vi "CLD 10 Step Sequencer with CSV Solution.vi"() -> ()   [LabVIEW 2014]
doc: "CLD-Übung 10\n\nDurch Verwendung des Zustandsautomaten aus CLD 9 und der FGV aus CLD-Übung 6 lässt sich die Entwicklungszeit für diese Übung verkürzen."
uses:
  CLD 10 CSV file read eum.ctl
  CLD 10 CSV file data structure.ctl
  CLD 10 CSV file enum.ctl
panel:
  out "Dauer des aktuellen Schritts":dbl
  out "Verstrichene Zeit (s)":dbl format="%#.2g"
  out "Schritt 3":bool
  out "Schritt 2":bool
  out "Schritt 1":bool
  out "Zeit ist verstrichen":bool
  in  "Autom. zurücksetzen":bool=TRUE
  in  "Zurücksetzen-Schaltfläche":bool
  in  "VI anhalten":bool
  out "Fehler (Ausgang)":errorcluster
  in  "Fehler (Eingang, kein Fehler)":errorcluster
  in  "Zielzeit (s)":dbl
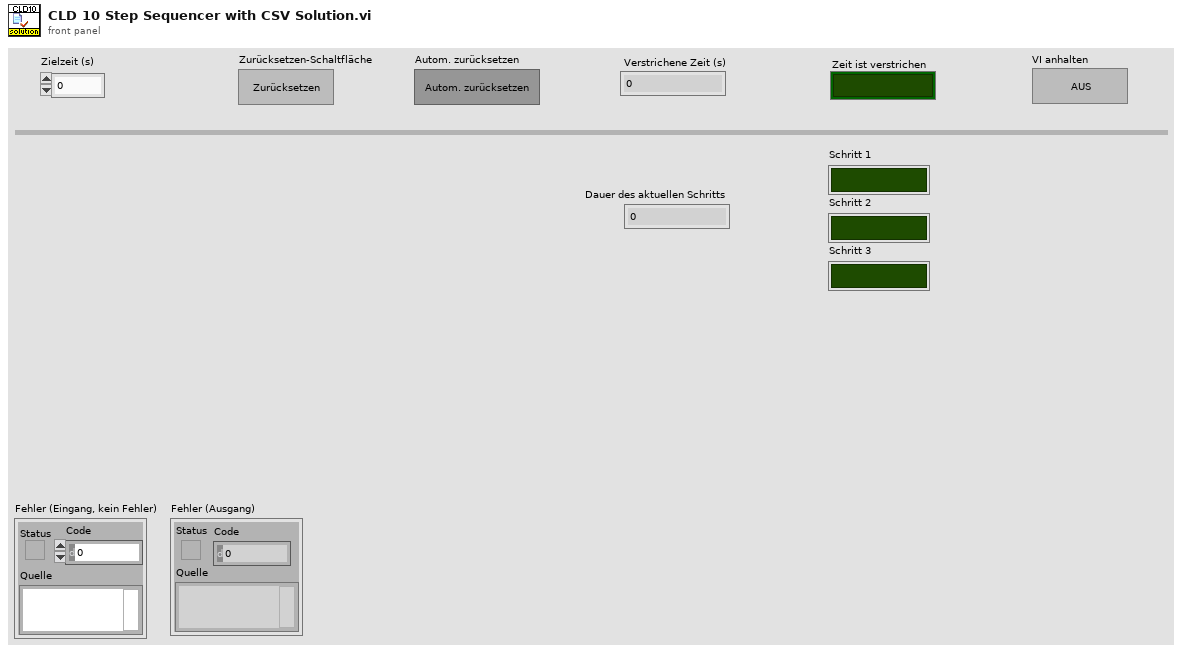
[diagram p1: front panel]
types:
  T1 = typedef "CLD 10 CSV file data structure.ctl" = cluster{"Schrittdauer - Ziel":i32, "Schritt 1":bool, "Schritt 2":bool, "Schritt 3":bool}
  T2 = typedef "CLD 10 CSV file read eum.ctl" = enum16{"CSV-Datei lesen", "Schritt eins ausführen", "Schritt zwei ausführen", "Schritt drei ausführen"}
  T3 = typedef "CLD 10 CSV file enum.ctl" = enum16{"CSV lesen", "CSV schreiben"}
  T4 = cluster{"Status":bool, "Code":i32, "Quelle":string}
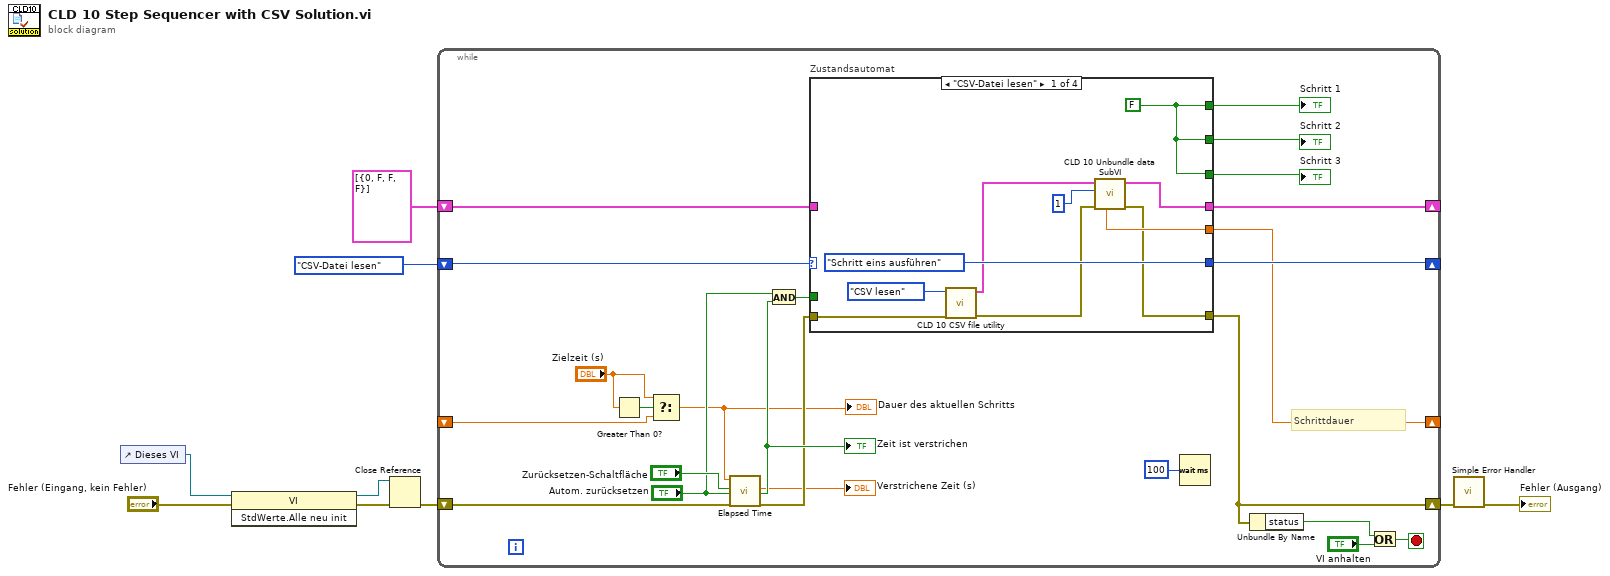
[diagram p0: block diagram]
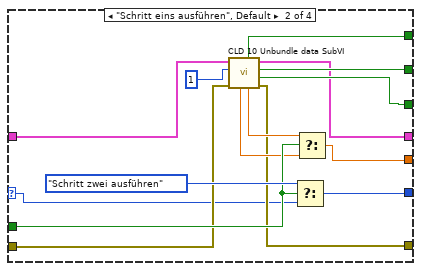
[diagram p2: hidden frame]
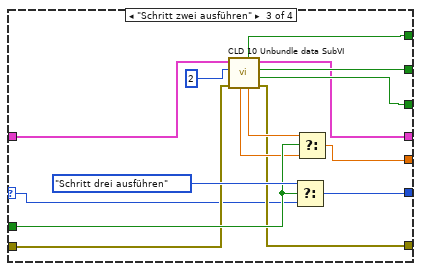
[diagram p3: hidden frame]
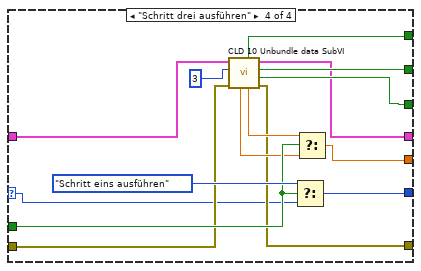
[diagram p4: hidden frame]
diagram:
  n1 = control-ref of="Dieses VI"() -> (w6:refnum<vi>)
  n2 = invoke on="Invoke Node" class="VI" method="StdWerte.Alle neu init"(reference=w6, error in="Fehler (Eingang, kein Fehler)") -> (reference out=w4:refnum<vi>, error out=w7:errorcluster)  [unwired: 1 in, 1 out]
  n3 = Close Reference(reference=w4, error in (no error)=w7) -> (error out=w5:errorcluster)
  n4 = while {
    shift-right: [w11] -> w8
    shift-left: w5 -> [w31]
    shift-right: [w29] -> _
    shift-left: CLD_10_CSV_file_read_eum."CSV-Datei lesen" ("Enum") -> [w28]
    shift-right: [w21] -> _
    shift-left: _ -> [w20]
    shift-right: [w15] -> _
    shift-left: T1[] [{"Schrittdauer - Ziel"=0, "Schritt 1"=FALSE, "Schritt 2"=FALSE, "Schritt 3"=FALSE}] ("[Daten, Ausgang]") -> [w14]
    stop <- w17 stop-if-true
    # "Schrittdauer"
    n5 = Greater Than 0?(x="Zielzeit (s)") -> (x > 0?=w23:bool)
    n6 = Select(t="Zielzeit (s)", s=w23, f=w20) -> (s? t:f=w12:dbl)
    "Dauer des aktuellen Schritts" <- w12
    n7 = call "Elapsed Time"("Time Target (s)"=w12, "Reset"="Zurücksetzen-Schaltfläche", "Auto Reset"="Autom. zurücksetzen", "error in (no error)"=w31) -> ("Elapsed Time (s)"=→"Verstrichene Zeit (s)":dbl, "Time has Elapsed"=w27:bool, "error out"=w13:errorcluster)  [unwired: 8 in, 5 out]
    "Zeit ist verstrichen" <- w27
    n8 = And(x="Autom. zurücksetzen", y=w27) -> (x .and. y?=w19:bool)
    n9 = case "Zustandsautomat" shown="\"CSV-Datei lesen\"" w28 {
      selector: w28 -> [_ w46 w61 w76]
      tunnel: [CLD_10_CSV_file_read_eum."Schritt eins ausführen" ("Enum") w57 w72 w87] -> w29
      tunnel: w19 -> [_ w56 w71 w86]
      tunnel: [w42 w45 w60 w75] -> w26
      tunnel: [w42 w50 w65 w80] -> w25
      tunnel: [w42 w49 w64 w79] -> w24
      tunnel: [w37 w55 w70 w85] -> w21
      tunnel: [w36 w44 w59 w74] -> w15
      tunnel: w14 -> [_ w54 w69 w84]
      tunnel: w13 -> [w40 w48 w63 w78]
      tunnel: [w34 w47 w62 w77] -> w11
      frame "CSV-Datei lesen" {
        w42 = FALSE
        n10 = call "CLD 10 CSV file utility.vi"("Fehler (Eingang)"=w40, "CSV-Datei-Enum"=CLD_10_CSV_file_enum."CSV lesen") -> ("Fehler (Ausgang)"=w35:T4, "[Daten, Ausgang]"=w39:T1[])  [unwired: 8 in]
        n11 = call "CLD 10 Unbundle data SubVI.vi"("Fehler (Eingang, kein Fehler)"=w35, "Nr. des aktuellen Zustands"=1 ("Nummer des Zustands"), "[Daten, Eingang]"=w39) -> ("Fehler (Ausgang)"=w34:errorcluster, "[Daten, Ausgang]"=w36:T1[], "Verweildauer"=w37:dbl)  [unwired: 2 in, 4 out]
      }
      frame "Schritt eins ausführen", Default {
        n12 = call "CLD 10 Unbundle data SubVI.vi"("Fehler (Eingang, kein Fehler)"=w48, "Nr. des aktuellen Zustands"=1 ("Nummer des Zustands"), "[Daten, Eingang]"=w54) -> ("Fehler (Ausgang)"=w47:errorcluster, "Zustand 3"=w49:bool, "Zustand 2"=w50:bool, "[Daten, Ausgang]"=w44:T1[], "Nächste Verweildauer"=w52:dbl, "Zustand 1"=w45:bool, "Verweildauer"=w51:dbl)  [unwired: 2 in]
        n13 = Select(t=CLD_10_CSV_file_read_eum."Schritt zwei ausführen" ("CLD 10 - Timer-Enum"), s=w56, f=w46) -> (s? t:f=w57:T2)
        n14 = Select(t=w52, s=w56, f=w51) -> (s? t:f=w55:dbl)
      }
      frame "Schritt zwei ausführen" {
        n15 = call "CLD 10 Unbundle data SubVI.vi"("Fehler (Eingang, kein Fehler)"=w63, "Nr. des aktuellen Zustands"=2 ("Nummer des Zustands"), "[Daten, Eingang]"=w69) -> ("Fehler (Ausgang)"=w62:errorcluster, "Zustand 3"=w64:bool, "Zustand 2"=w65:bool, "[Daten, Ausgang]"=w59:T1[], "Nächste Verweildauer"=w67:dbl, "Zustand 1"=w60:bool, "Verweildauer"=w66:dbl)  [unwired: 2 in]
        n16 = Select(t=CLD_10_CSV_file_read_eum."Schritt drei ausführen" ("CLD 10 - Timer-Enum"), s=w71, f=w61) -> (s? t:f=w72:T2)
        n17 = Select(t=w67, s=w71, f=w66) -> (s? t:f=w70:dbl)
      }
      frame "Schritt drei ausführen" {
        n18 = call "CLD 10 Unbundle data SubVI.vi"("Fehler (Eingang, kein Fehler)"=w78, "Nr. des aktuellen Zustands"=3 ("Nummer des Zustands"), "[Daten, Eingang]"=w84) -> ("Fehler (Ausgang)"=w77:errorcluster, "Zustand 3"=w79:bool, "Zustand 2"=w80:bool, "[Daten, Ausgang]"=w74:T1[], "Nächste Verweildauer"=w82:dbl, "Zustand 1"=w75:bool, "Verweildauer"=w81:dbl)  [unwired: 2 in]
        n19 = Select(t=CLD_10_CSV_file_read_eum."Schritt eins ausführen" ("CLD 10 - Timer-Enum"), s=w86, f=w76) -> (s? t:f=w87:T2)
        n20 = Select(t=w82, s=w86, f=w81) -> (s? t:f=w85:dbl)
      }
    }
    "Schritt 1" <- w26
    "Schritt 2" <- w25
    "Schritt 3" <- w24
    n21 = Wait (ms)(milliseconds to wait=u32 100 ("Zu wartende ms")) -> ()  [unwired: 1 out]
    n22 = Unbundle By Name(w11) -> ("status"=w16:bool)
    n23 = Or(x=w16, y="VI anhalten") -> (x .or. y?=w17:bool)
  }
  n24 = call <vilib>:"Simple Error Handler.vi"("error in (no error)"=w8) -> ("error out"=→"Fehler (Ausgang)":errorcluster)  [unwired: 4 in, 4 out]
